vi "_7Case_Structures2.vi"() -> ()   [LabVIEW 2018]
panel:
  out "Day":string
  in  "Day Number":dbl
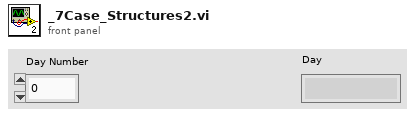
[diagram p1: front panel]
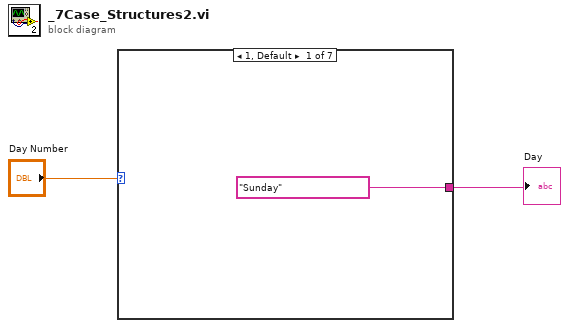
[diagram p0: block diagram]
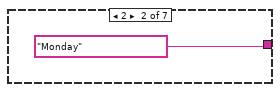
[diagram p2: hidden frame]
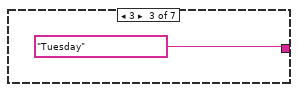
[diagram p3: hidden frame]
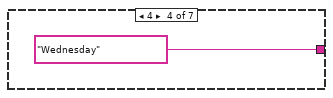
[diagram p4: hidden frame]
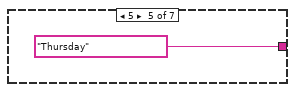
[diagram p5: hidden frame]
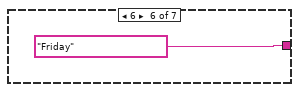
[diagram p6: hidden frame]
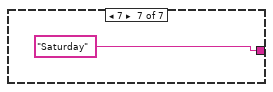
[diagram p7: hidden frame]
diagram:
  n1 = case shown="1, Default" "Day Number" {
    tunnel: ["Sunday" "Monday" "Tuesday" "Wednesday" "Thursday" "Friday" "Saturday"] -> w2
    frame 1, Default {
    }
    frame 2 {
    }
    frame 3 {
    }
    frame 4 {
    }
    frame 5 {
    }
    frame 6 {
    }
    frame 7 {
    }
  }
  "Day" <- w2
